vi "niScope Clear Waveform Processing.vi"(0 "instrument handle":refnum<k15>, 5 "channels":string="0", 11 "error in":errorcluster) -> (4 "instrument handle out":refnum<k15>, 15 "error out":errorcluster)   [LabVIEW 2011]
doc: "Clears the list of processing steps assigned to the given channel."
uses:
  niScope_32.dll
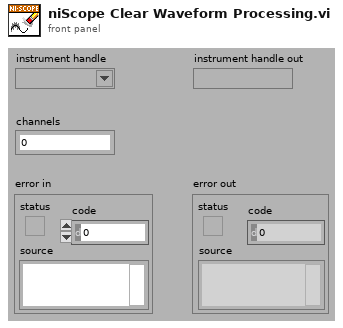
[diagram p1: front panel]
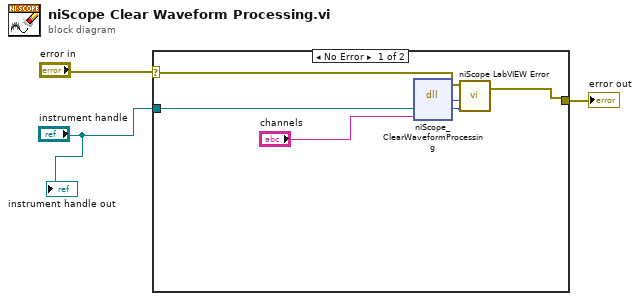
[diagram p0: block diagram]
diagram:
  n1 = case shown="No Error" "error in" {
    selector: "error in" -> [w4 w10]
    tunnel: [w5 w10] -> w2
    tunnel: "instrument handle" -> [w9 _]
    frame No Error {
      n2 = dll-call lib="niScope_*.*" fn="niScope_ClearWaveformProcessing"("instrument handle"=w9, "channel"="channels") -> ("status"=w7:i32, "instrument handle"=w6:u32)  [unwired: 4 in, 2 out]
      n3 = call <instrlib>:"niScope LabVIEW Error.vi"("instrument handle"=w6, "niScope error code (0)"=w7, "error in (no error)"=w4) -> ("error out"=w5:errorcluster)  [unwired: 2 in]
    }
    frame Error {
    }
  }
  "error out" <- w2
  "instrument handle out" <- "instrument handle"
